vi "Base Init.vi"(9 "Actor":refnum<class "Actor.lvclass">, 10 "Self Alias":string) -> (2 "Actor":refnum<class "Actor.lvclass">)   [LabVIEW 2021, in "jettl.lvlib" / "Temporary Actor.lvlib"]
uses:
  Temporary Actor.lvlib
  Addresses Strategy/Addresses Strategy.lvlib
  jettl Actor/jettl Actor.lvclass
  Msg/Msg.lvclass
  C:/git/jettl/jettl/jettl/Temporary Actor/Actor/Actor.lvclass
  C:/git/jettl/jettl/jettl/Last Ack Msg/Last Ack/Last Ack.lvclass
  C:/git/jettl/jettl/jettl/Setup Msg/Setup/Setup.lvclass
  C:/git/jettl/jettl/jettl/Teardown Msg/Teardown/Teardown.lvclass
  C:/git/jettl/jettl/jettl/Temporary Actor/jettl Actor/jettl Actor.lvclass
  Actor/Actor.lvclass
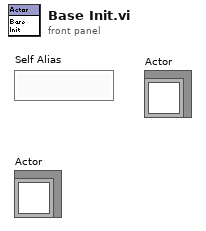
[diagram p1: front panel]
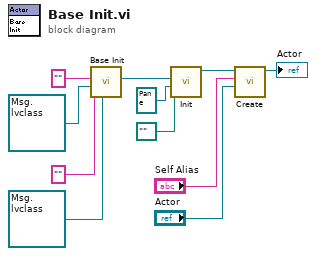
[diagram p0: block diagram]
diagram:
  n1 = call "Base Init.vi"("Creator"=refnum<user-event> refnum, "Creator Alias"="", "Self"=refnum<user-event> refnum, "Self Alias"="") -> ("Addresses Strategy out"=w7:refnum<class "Addresses Strategy.lvclass">)  [unwired: 7 in]
  n2 = call "Init.vi"("Path"=path "", "Register"=refnum<event-registration> refnum, "Addresses Strategy"=w7) -> ("jettl Actor out"=w8:refnum<class "jettl Actor.lvclass">)  [unwired: 8 in]
  n3 = call-dynamic "Create.vi"("Actor"="Actor", "Self Alias"="Self Alias", "jettl Actor in"=w8) -> ("jettl Actor out"=→"Actor":refnum<class "jettl Actor.lvclass">)  [unwired: 8 in]
